vi "drive-auto.vi"() -> ()   [LabVIEW 2018]
doc: "This VI is called for each TeleOp packet received from the DS where the robot is not disabled. It is often used to read from the joysticks and update I/O or to update setpoints for timed control loops. It should complete and return within 20 milliseconds or it may miss DS packets."
uses:
  <vilib>/Rock Robotics/WPI/Solenoid/WPI_SolenoidValue.ctl
  <vilib>/Rock Robotics/WPI/ThirdParty/Phoenix-LabVIEW/Motor Controller/Controls/CTRE_Phoenix_MotorControl_ControlMode.ctl
  2e9e096c-a0d6-4374-a758-daa4b7bc34b9.vi
  069bde93-6a50-4702-a448-63a100da85ba.vi
  93fe4f39-d887-44e8-b42b-40b0db67de57.vi
  <vilib>/Rock Robotics/WPI/Utilities/WPI_GetSetVariantRefNum.vi
  <vilib>/Rock Robotics/Network Tables/NT Write Boolean Array.vi
  <vilib>/Rock Robotics/Network Tables/NT Write Numeric Array.vi
  Robot Global Data.vi
  <vilib>/Rock Robotics/WPI/Solenoid/WPI_SolenoidSetEnum.vi
  <vilib>/Rock Robotics/WPI/ThirdParty/Phoenix-LabVIEW/Motor Controller/Get/CTRE_Phoenix_MotorController_GetSelectedSensorData.vi
  <vilib>/Rock Robotics/WPI/ThirdParty/Phoenix-LabVIEW/Motor Controller/Get/CTRE_Phoenix_MotorController_GetOutputCurrent_Enhanced.vi
panel:
  out "Level":string="Low"
  out "GamePiece":string="Hatch"
  out "Output Voltage 4":dbl
  out "Output Voltage 3":dbl
  out "Output Voltage 2":dbl
  out "Output Voltage":dbl
  out "wrist sensor":i32
  out "Arm sensor":i32
  out "x output 2":dbl
  out "y output 2":dbl
  # "left"
  # "RIGHT"
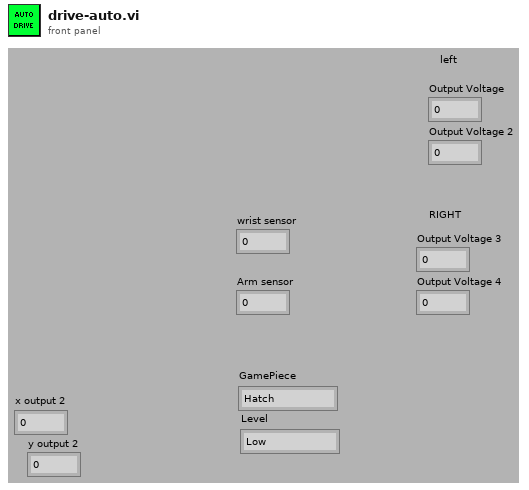
[diagram p1: front panel]
types:
  T1 = typedef "WPI_SolenoidValue.ctl" = enum16{"Off", "On", "Forward", "Reverse"}
  T2 = typedef "WPI_JoystickDevRef.ctl" = cluster{"Device":T3}
  T3 = typedef "WPI_JoystickDeviceEnum.ctl" = enum16{"USB 0", "USB 1", "USB 2", "USB 3", "USB 4", "USB 5"}
  T4 = typedef "WPI_RobotDriveDevRef.ctl" = cluster{"DevStatus":errorcluster, "Motors[]":T5[], "Square Inputs":bool, "Max Output":dbl}
  T5 = typedef "WPI_MotorControlDeviceRef.ctl" = cluster{"DeviceStatus":errorcluster, "Type":T6, "PWM":cluster{"PWM Channel":T7, "DeadBand":T8}, "CAN":cluster{"Device Number":u8, "SetOutput VI Ref":variant, "GetOutput VI Ref":variant, "Enable VI Ref":variant, "Disable VI Ref":variant, "Data":variant}, "Invert":bool, "DIO PWM":cluster{"PWM \"Enable\" Channel":T7, "DIOChannel":T9, "PWM Rate":dbl}}
  T6 = typedef "WPI_MotorControlType.ctl" = enum16{"PWM", "CAN", "DIO PWM"}
  T7 = typedef "FPGA_DIOPWMChannel.ctl" = enum8{"PWM 0", "PWM 1", "PWM 2", "PWM 3", "PWM 4", "PWM 5", "PWM 6", "PWM 7", "PWM 8", "PWM 9", "PWM MXP 0", "PWM MXP 1", "PWM MXP 2", "PWM MXP 3", "PWM MXP 4", "PWM MXP 5", "PWM MXP 6", "PWM MXP 7", "PWM MXP 8", "PWM MXP 9", "Invalid"}
  T8 = typedef "WPI_PWMDeadband.ctl" = cluster{"Name":string, "maxPositivePwm":i32, "minPositivePwm":i32, "centerPwm":i32, "maxNegativePwm":i32, "minNegativePwm":i32, "angularRange":u16}
  T9 = typedef "FPGA_DIOChannel.ctl" = enum8{"DIO 0", "DIO 1", "DIO 2", "DIO 3", "DIO 4", "DIO 5", "DIO 6", "DIO 7", "DIO 8", "DIO 9", "DIO MXP 0", "DIO MXP 1", "DIO MXP 2", "DIO MXP 3", "DIO MXP 4", "DIO MXP 5", "DIO MXP 6", "DIO MXP 7", "DIO MXP 8", "DIO MXP 9", "DIO MXP 10", "DIO MXP 11", "DIO MXP 12", "DIO MXP 13", "DIO MXP 14", "DIO MXP 15", "SPI Port CS1", "SPI Port CS2", "SPI Port CS3", "SPI Port MISO", "SPI Port MOSI", "Invalid"}
  T10 = typedef "WPI_SolenoidDevRef.ctl" = cluster{"DevStatus":errorcluster, "Pneumatics Control Module":u8, "Forward Solenoid Channel":T11, "Reverse Solenoid Channel":T11}
  T11 = typedef "WPI_SolenoidChannel.ctl" = enum8{"Solenoid 0", "Solenoid 1", "Solenoid 2", "Solenoid 3", "Solenoid 4", "Solenoid 5", "Solenoid 6", "Solenoid 7", "Invalid"}
  T12 = typedef "CTRE_Phoenix_MotorControl_ControlMode.ctl" = u16
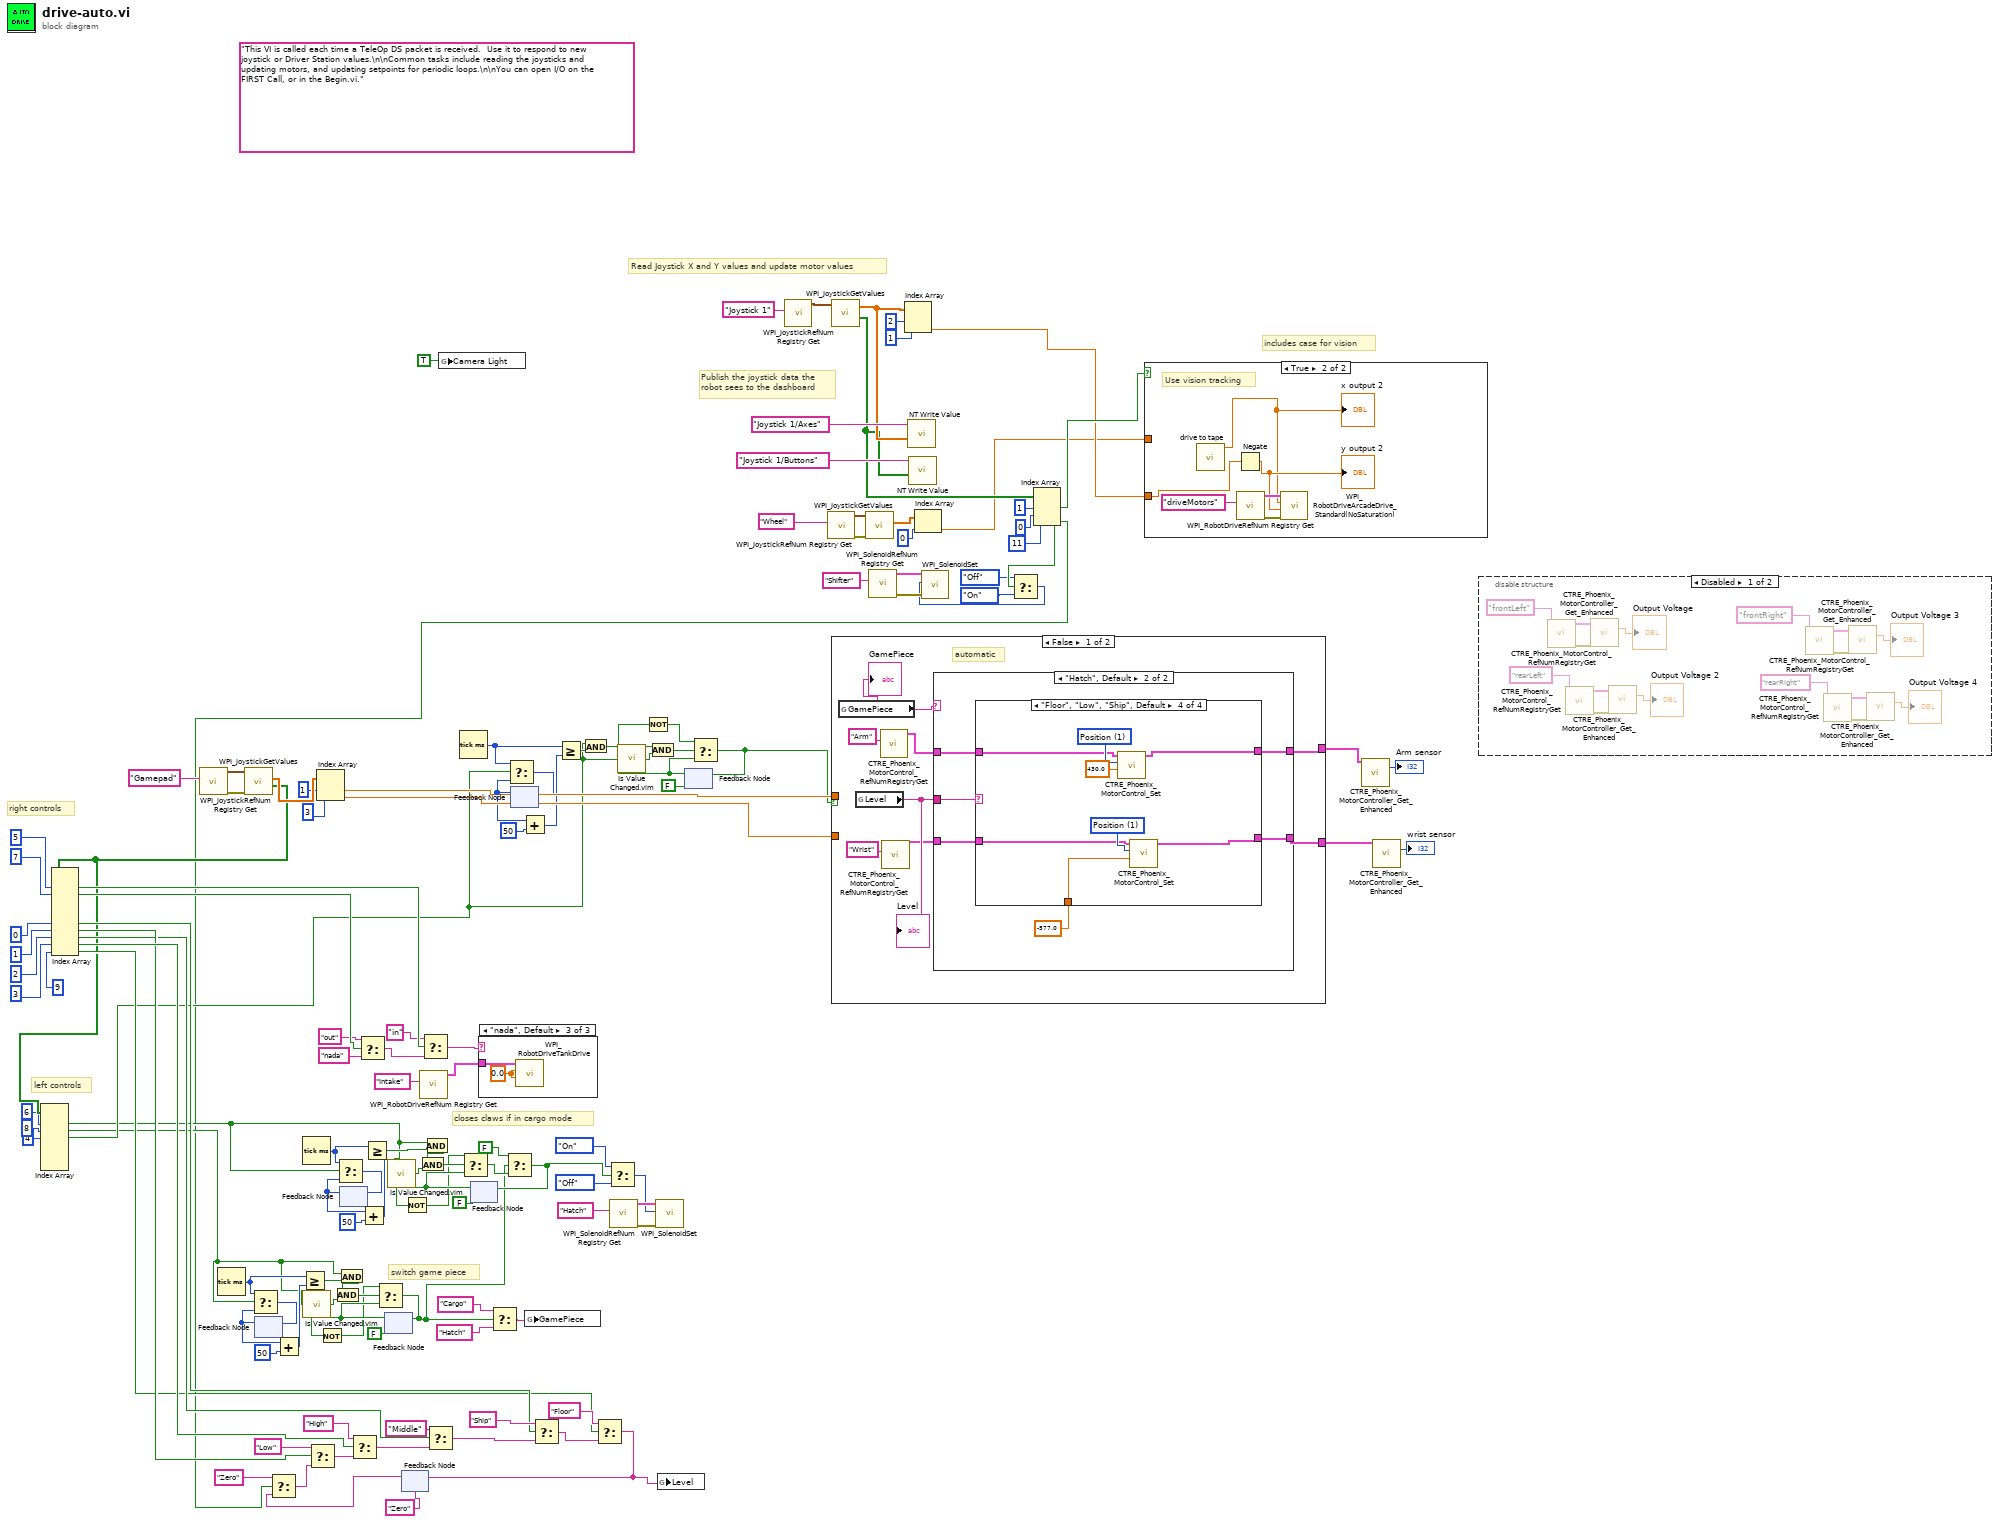
[diagram p0: block diagram]
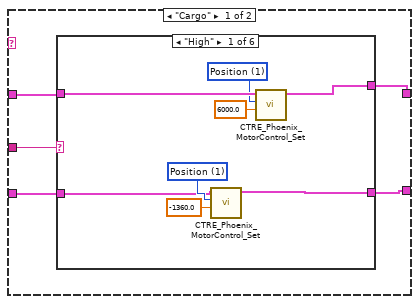
[diagram p3: hidden frame]
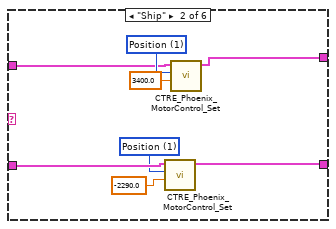
[diagram p4: hidden frame]
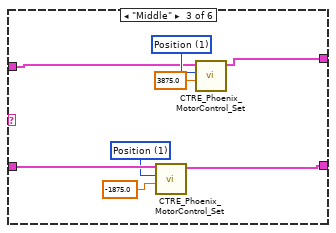
[diagram p5: hidden frame]
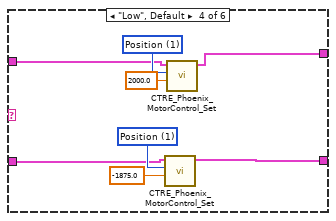
[diagram p6: hidden frame]
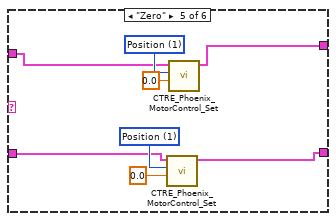
[diagram p7: hidden frame]
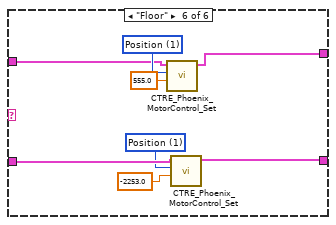
[diagram p8: hidden frame]
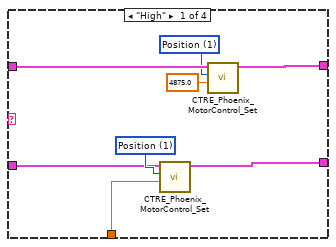
[diagram p9: hidden frame]
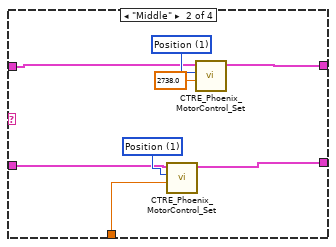
[diagram p10: hidden frame]
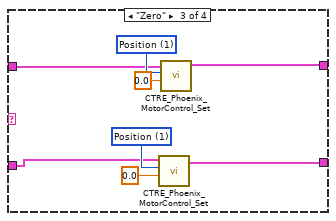
[diagram p11: hidden frame]
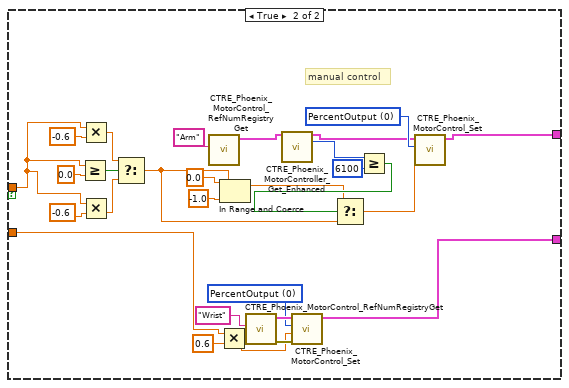
[diagram p12: hidden frame]
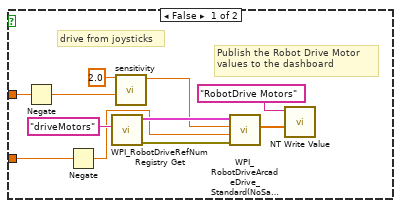
[diagram p13: hidden frame]
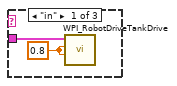
[diagram p14: hidden frame]
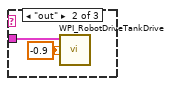
[diagram p15: hidden frame]
diagram:
  (unwired) "This VI is called each time a TeleOp DS packet is received.  Use it to respond to new joystick or Driver Station values.\n\nCommon tasks include reading the joysticks and updating motors, and updating setpoints for periodic loops.\n\nYou can open I/O on the FIRST Call, or in the Begin.vi."
  # "closes claws if in cargo mode"
  # "switch game piece"
  # "left controls"
  # "right controls"
  # "includes case for vision"
  # "Publish the joystick data the\nrobot sees to the dashboard"
  # "Read Joystick X and Y values and update motor values"
  n1 = call <vilib>:"WPI_JoystickRefNum Registry Get.vi"("refnum name"="Gamepad") -> ("error out"=w114:errorcluster, "JoystickDevRef"=w117:T2)  [unwired: 1 in, 8 out]
  n2 = Tick Count (ms)() -> (millisecond timer value=w49:u32)
  n3 = call <vilib>:"WPI_JoystickGetValues.vi"("error in (no error)"=w114, "JoystickDevRef"=w117) -> ("Buttons"=w18:bool[], "Axes"=w116:dbl[])  [unwired: 5 in, 3 out]
  n4 = Index Array(array=w18, index #1=6 ("index"), index #2=8 ("index"), index #3=4 ("index")) -> (element #1=w12:bool, element #2=w13:bool, element #3=w14:bool)  [unwired: 4 in, 4 out]
  n5 = Index Array(array=w18, index #1=5 ("index"), index #2=7 ("index"), index #6=0 ("index"), index #7=1 ("index"), index #8=2 ("index"), index #9=3 ("index"), index #10=9 ("index")) -> (element #1=w111:bool, element #2=w106:bool, element #6=w25:bool, element #7=w24:bool, element #8=w23:bool, element #9=w26:bool, element #10=w19:bool)  [unwired: 3 in, 3 out]
  n6 = feedback #1() -> (w40:u32)  [unwired: 1 in]
  n7 = Select(t=w49, s=w13, f=w40) -> (s? t:f=w47:u32)
  n8 = feedback-in #1(w47) -> ()
  n9 = Add(x=w40, y=u32 50) -> (x+y=w48:u32)
  n10 = Greater Or Equal?(x=w49, y=w48) -> (x >= y?=w50:bool)
  n11 = Tick Count (ms)() -> (millisecond timer value=w81:u32)
  n12 = call "Is Value Changed.vim"("value"=w13) -> ("changed or first call?"=w45:bool)
  n13 = Index Array(array=w116, index #1=1 ("index"), index #2=3 ("index")) -> (element #1=w70:dbl, element #2=w71:dbl)
  n14 = And(x=w13, y=w50) -> (x .and. y?=w51:bool)
  n15 = And(x=w51, y=w45) -> (x .and. y?=w44:bool)
  n16 = feedback #2() -> (w72:u32)  [unwired: 1 in]
  n17 = Select(t=w81, s=w12, f=w72) -> (s? t:f=w79:u32)
  n18 = feedback-in #2(w79) -> ()
  n19 = Select(t="out", s=w106, f="nada") -> (s? t:f=w107:string)
  n20 = Add(x=w72, y=u32 50) -> (x+y=w80:u32)
  n21 = Greater Or Equal?(x=w81, y=w80) -> (x >= y?=w82:bool)
  n22 = feedback #3(FALSE) -> (w43:bool)
  n23 = Not(x=w43) -> (.not. x?=w41:bool)
  n24 = Select(t=w41, s=w44, f=w43) -> (s? t:f=w2:bool)
  n25 = feedback-in #3(w2) -> ()
  n26 = call "Is Value Changed.vim"("value"=w12) -> ("changed or first call?"=w77:bool)
  n27 = feedback #4("Zero") -> (w9:string)
  n28 = call <vilib>:"WPI_RobotDriveRefNum Registry Get.vi"("refnum name"="Intake") -> ("RobotDriveDevRef"=w102:T4)  [unwired: 9 in, 1 out]
  n29 = Select(t="in", s=w111, f=w107) -> (s? t:f=w110:string)
  n30 = And(x=w12, y=w82) -> (x .and. y?=w83:bool)
  n31 = And(x=w83, y=w77) -> (x .and. y?=w76:bool)
  n32 = global write "Robot Global Data.vi" "Camera Light"(TRUE ("Camera Light")) -> ()
  n33 = Tick Count (ms)() -> (millisecond timer value=w67:u32)
  n34 = feedback #5(FALSE) -> (w75:bool)
  n35 = Not(x=w75) -> (.not. x?=w73:bool)
  n36 = Select(t=w73, s=w76, f=w75) -> (s? t:f=w3:bool)
  n37 = case shown="\"nada\", Default" w110 {
    tunnel: w102 -> [w133 w135 w137]
    frame "in" {
      w134 = 0.8
      n38 = call <vilib>:"WPI_RobotDriveTankDrive.vi"("Right axis value"=w134, "Left axis value"=w134, "RobotDriveDevRef"=w133) -> ()  [unwired: 6 in, 3 out]
    }
    frame "out" {
      w136 = -0.9
      n39 = call <vilib>:"WPI_RobotDriveTankDrive.vi"("Right axis value"=w136, "Left axis value"=w136, "RobotDriveDevRef"=w135) -> ()  [unwired: 6 in, 3 out]
    }
    frame "nada", Default {
      w138 = 0.0
      n40 = call <vilib>:"WPI_RobotDriveTankDrive.vi"("Right axis value"=w138, "Left axis value"=w138, "RobotDriveDevRef"=w137) -> ()  [unwired: 6 in, 3 out]
    }
  }
  n41 = Select(t="Cargo", s=w2, f="Hatch") -> (s? t:f=w53:string)
  n42 = Select(t=FALSE, s=w2, f=w3) -> (s? t:f=w4:bool)
  n43 = feedback-in #5(w4) -> ()
  n44 = feedback #6() -> (w58:u32)  [unwired: 1 in]
  n45 = Select(t=w67, s=w14, f=w58) -> (s? t:f=w65:u32)
  n46 = feedback-in #6(w65) -> ()
  n47 = Add(x=w58, y=u32 50) -> (x+y=w66:u32)
  n48 = global write "Robot Global Data.vi" "GamePiece"(w53) -> ()
  n49 = Greater Or Equal?(x=w67, y=w66) -> (x >= y?=w68:bool)
  n50 = And(x=w14, y=w68) -> (x .and. y?=w69:bool)
  n51 = Select(t=WPI_SolenoidValue."On" ("Value"), s=w4, f=WPI_SolenoidValue."Off") -> (s? t:f=w98:T1)
  n52 = call <vilib>:"WPI_SolenoidRefNum Registry Get.vi"("refnum name"="Hatch") -> ("error out"=w101:errorcluster, "SolenoidDevRef"=w100:T10)  [unwired: 9 in]
  n53 = call "Is Value Changed.vim"("value"=w14) -> ("changed or first call?"=w63:bool)
  n54 = And(x=w69, y=w63) -> (x .and. y?=w62:bool)
  n55 = call-poly <vilib>:"WPI_SolenoidSet.vi"("error in (no error)"=w101, "Value"=w98, "SolenoidDevRef"=w100) -> ()  [unwired: 7 in, 2 out]
  n56 = feedback #7(FALSE) -> (w61:bool)
  n57 = Not(x=w61) -> (.not. x?=w59:bool)
  n58 = Select(t=w59, s=w62, f=w61) -> (s? t:f=w57:bool)
  n59 = feedback-in #7(w57) -> ()
  n60 = call <vilib>:"WPI_JoystickRefNum Registry Get.vi"("refnum name"="Joystick 1") -> ("JoystickDevRef"=w131:T2)  [unwired: 1 in, 9 out]
  n61 = call <vilib>:"WPI_JoystickRefNum Registry Get.vi"("refnum name"="Wheel") -> ("error out"=w125:errorcluster, "JoystickDevRef"=w124:T2)  [unwired: 9 in]
  n62 = call <vilib>:"WPI_JoystickGetValues.vi"("JoystickDevRef"=w131) -> ("Buttons"=w120:bool[], "Axes"=w128:dbl[])  [unwired: 6 in, 3 out]
  n63 = case shown="False" w57 {
    tunnel: w71 -> [_ w258]
    tunnel: w70 -> [_ w250]
    tunnel: [w139 w249] -> w55
    tunnel: [w143 w248] -> w54
    frame False {
      # "automatic"
      n64 = global read "Robot Global Data.vi" "GamePiece"() -> (w142:string)
      "GamePiece" <- w142
      n65 = global read "Robot Global Data.vi" "Level"() -> (w141:string)
      "Level" <- w141
      n66 = call <vilib>:"CTRE_Phoenix_MotorControl_RefNumRegistryGet.vi"("refnum name"="Arm") -> ("PhoenixMotorControlDevRef"=w146:T5)  [unwired: 9 in, 1 out]
      n67 = call <vilib>:"CTRE_Phoenix_MotorControl_RefNumRegistryGet.vi"("refnum name"="Wrist") -> ("PhoenixMotorControlDevRef"=w140:T5)  [unwired: 9 in, 1 out]
      n68 = case shown="\"Hatch\", Default" w142 {
        tunnel: w146 -> [w150 w205]
        tunnel: [w151 w204] -> w143
        tunnel: [w149 w203] -> w139
        tunnel: w141 -> [w148 w202]
        tunnel: w140 -> [w147 w201]
        frame "Cargo" {
          n69 = case shown="\"High\"" w148 {
            tunnel: w150 -> [w159 w166 w174 w182 w187 w198]
            tunnel: [w157 w165 w173 w181 w186 w197] -> w151
            tunnel: [w155 w163 w171 w179 w185 w195] -> w149
            tunnel: w147 -> [w152 w162 w170 w176 w184 w194]
            frame "High" {
              w153 = T12 1 items=["PercentOutput"=0, "Position"=1, "Velocity"=2, "Current"=3, "Follower"=5, "MotionProfile"=6, "MotionMagic"=7, "MotionProfileArc"=10, "Disabled"=15] ("Control Mode")
              w158 = T12 1 items=["PercentOutput"=0, "Position"=1, "Velocity"=2, "Current"=3, "Follower"=5, "MotionProfile"=6, "MotionMagic"=7, "MotionProfileArc"=10, "Disabled"=15] ("Control Mode")
              n70 = call <vilib>:"CTRE_Phoenix_MotorControl_Set.vi"("Output"=-1360.0, "Control Mode"=w153, "PhoenixMotorControlDevRef"=w152) -> ("PhoenixMotorControlDevRef"=w155:T5)  [unwired: 7 in, 1 out]
              n71 = call <vilib>:"CTRE_Phoenix_MotorControl_Set.vi"("Output"=6000.0, "Control Mode"=w158, "PhoenixMotorControlDevRef"=w159) -> ("PhoenixMotorControlDevRef"=w157:T5)  [unwired: 7 in, 1 out]
            }
            frame "Ship" {
              w160 = T12 1 items=["PercentOutput"=0, "Position"=1, "Velocity"=2, "Current"=3, "Follower"=5, "MotionProfile"=6, "MotionMagic"=7, "MotionProfileArc"=10, "Disabled"=15] ("Control Mode")
              w167 = T12 1 items=["PercentOutput"=0, "Position"=1, "Velocity"=2, "Current"=3, "Follower"=5, "MotionProfile"=6, "MotionMagic"=7, "MotionProfileArc"=10, "Disabled"=15] ("Control Mode")
              n72 = call <vilib>:"CTRE_Phoenix_MotorControl_Set.vi"("Output"=-2290.0, "Control Mode"=w160, "PhoenixMotorControlDevRef"=w162) -> ("PhoenixMotorControlDevRef"=w163:T5)  [unwired: 7 in, 1 out]
              n73 = call <vilib>:"CTRE_Phoenix_MotorControl_Set.vi"("Output"=3400.0, "Control Mode"=w167, "PhoenixMotorControlDevRef"=w166) -> ("PhoenixMotorControlDevRef"=w165:T5)  [unwired: 7 in, 1 out]
            }
            frame "Middle" {
              w168 = T12 1 items=["PercentOutput"=0, "Position"=1, "Velocity"=2, "Current"=3, "Follower"=5, "MotionProfile"=6, "MotionMagic"=7, "MotionProfileArc"=10, "Disabled"=15] ("Control Mode")
              w175 = T12 1 items=["PercentOutput"=0, "Position"=1, "Velocity"=2, "Current"=3, "Follower"=5, "MotionProfile"=6, "MotionMagic"=7, "MotionProfileArc"=10, "Disabled"=15] ("Control Mode")
              n74 = call <vilib>:"CTRE_Phoenix_MotorControl_Set.vi"("Output"=-1875.0, "Control Mode"=w168, "PhoenixMotorControlDevRef"=w170) -> ("PhoenixMotorControlDevRef"=w171:T5)  [unwired: 7 in, 1 out]
              n75 = call <vilib>:"CTRE_Phoenix_MotorControl_Set.vi"("Output"=3875.0, "Control Mode"=w175, "PhoenixMotorControlDevRef"=w174) -> ("PhoenixMotorControlDevRef"=w173:T5)  [unwired: 7 in, 1 out]
            }
            frame "Low", Default {
              w177 = T12 1 items=["PercentOutput"=0, "Position"=1, "Velocity"=2, "Current"=3, "Follower"=5, "MotionProfile"=6, "MotionMagic"=7, "MotionProfileArc"=10, "Disabled"=15] ("Control Mode")
              w183 = T12 1 items=["PercentOutput"=0, "Position"=1, "Velocity"=2, "Current"=3, "Follower"=5, "MotionProfile"=6, "MotionMagic"=7, "MotionProfileArc"=10, "Disabled"=15] ("Control Mode")
              n76 = call <vilib>:"CTRE_Phoenix_MotorControl_Set.vi"("Output"=-1875.0, "Control Mode"=w177, "PhoenixMotorControlDevRef"=w176) -> ("PhoenixMotorControlDevRef"=w179:T5)  [unwired: 7 in, 1 out]
              n77 = call <vilib>:"CTRE_Phoenix_MotorControl_Set.vi"("Output"=2000.0, "Control Mode"=w183, "PhoenixMotorControlDevRef"=w182) -> ("PhoenixMotorControlDevRef"=w181:T5)  [unwired: 7 in, 1 out]
            }
            frame "Zero" {
              w188 = T12 1 items=["PercentOutput"=0, "Position"=1, "Velocity"=2, "Current"=3, "Follower"=5, "MotionProfile"=6, "MotionMagic"=7, "MotionProfileArc"=10, "Disabled"=15] ("Control Mode")
              w191 = T12 1 items=["PercentOutput"=0, "Position"=1, "Velocity"=2, "Current"=3, "Follower"=5, "MotionProfile"=6, "MotionMagic"=7, "MotionProfileArc"=10, "Disabled"=15] ("Control Mode")
              n78 = call <vilib>:"CTRE_Phoenix_MotorControl_Set.vi"("Output"=0.0, "Control Mode"=w188, "PhoenixMotorControlDevRef"=w184) -> ("PhoenixMotorControlDevRef"=w185:T5)  [unwired: 7 in, 1 out]
              n79 = call <vilib>:"CTRE_Phoenix_MotorControl_Set.vi"("Output"=0.0, "Control Mode"=w191, "PhoenixMotorControlDevRef"=w187) -> ("PhoenixMotorControlDevRef"=w186:T5)  [unwired: 7 in, 1 out]
            }
            frame "Floor" {
              w192 = T12 1 items=["PercentOutput"=0, "Position"=1, "Velocity"=2, "Current"=3, "Follower"=5, "MotionProfile"=6, "MotionMagic"=7, "MotionProfileArc"=10, "Disabled"=15] ("Control Mode")
              w199 = T12 1 items=["PercentOutput"=0, "Position"=1, "Velocity"=2, "Current"=3, "Follower"=5, "MotionProfile"=6, "MotionMagic"=7, "MotionProfileArc"=10, "Disabled"=15] ("Control Mode")
              n80 = call <vilib>:"CTRE_Phoenix_MotorControl_Set.vi"("Output"=555.0, "Control Mode"=w199, "PhoenixMotorControlDevRef"=w198) -> ("PhoenixMotorControlDevRef"=w197:T5)  [unwired: 7 in, 1 out]
              n81 = call <vilib>:"CTRE_Phoenix_MotorControl_Set.vi"("Output"=-2253.0, "Control Mode"=w192, "PhoenixMotorControlDevRef"=w194) -> ("PhoenixMotorControlDevRef"=w195:T5)  [unwired: 7 in, 1 out]
            }
          }
        }
        frame "Hatch", Default {
          n82 = case shown="\"Floor\", \"Low\", \"Ship\", Default" w202 {
            tunnel: w205 -> [w213 w220 w225 w236]
            tunnel: [w211 w219 w224 w235] -> w204
            tunnel: [w209 w217 w223 w233] -> w203
            tunnel: w201 -> [w207 w215 w222 w231]
            tunnel: -577.0 ("Output") -> [w206 w214 _ w230]
            frame "High" {
              w208 = T12 1 items=["PercentOutput"=0, "Position"=1, "Velocity"=2, "Current"=3, "Follower"=5, "MotionProfile"=6, "MotionMagic"=7, "MotionProfileArc"=10, "Disabled"=15] ("Control Mode")
              w212 = T12 1 items=["PercentOutput"=0, "Position"=1, "Velocity"=2, "Current"=3, "Follower"=5, "MotionProfile"=6, "MotionMagic"=7, "MotionProfileArc"=10, "Disabled"=15] ("Control Mode")
              n83 = call <vilib>:"CTRE_Phoenix_MotorControl_Set.vi"("Output"=w206, "Control Mode"=w208, "PhoenixMotorControlDevRef"=w207) -> ("PhoenixMotorControlDevRef"=w209:T5)  [unwired: 7 in, 1 out]
              n84 = call <vilib>:"CTRE_Phoenix_MotorControl_Set.vi"("Output"=4875.0, "Control Mode"=w212, "PhoenixMotorControlDevRef"=w213) -> ("PhoenixMotorControlDevRef"=w211:T5)  [unwired: 7 in, 1 out]
            }
            frame "Middle" {
              w216 = T12 1 items=["PercentOutput"=0, "Position"=1, "Velocity"=2, "Current"=3, "Follower"=5, "MotionProfile"=6, "MotionMagic"=7, "MotionProfileArc"=10, "Disabled"=15] ("Control Mode")
              w221 = T12 1 items=["PercentOutput"=0, "Position"=1, "Velocity"=2, "Current"=3, "Follower"=5, "MotionProfile"=6, "MotionMagic"=7, "MotionProfileArc"=10, "Disabled"=15] ("Control Mode")
              n85 = call <vilib>:"CTRE_Phoenix_MotorControl_Set.vi"("Output"=w214, "Control Mode"=w216, "PhoenixMotorControlDevRef"=w215) -> ("PhoenixMotorControlDevRef"=w217:T5)  [unwired: 7 in, 1 out]
              n86 = call <vilib>:"CTRE_Phoenix_MotorControl_Set.vi"("Output"=2738.0, "Control Mode"=w221, "PhoenixMotorControlDevRef"=w220) -> ("PhoenixMotorControlDevRef"=w219:T5)  [unwired: 7 in, 1 out]
            }
            frame "Zero" {
              w226 = T12 1 items=["PercentOutput"=0, "Position"=1, "Velocity"=2, "Current"=3, "Follower"=5, "MotionProfile"=6, "MotionMagic"=7, "MotionProfileArc"=10, "Disabled"=15] ("Control Mode")
              w229 = T12 1 items=["PercentOutput"=0, "Position"=1, "Velocity"=2, "Current"=3, "Follower"=5, "MotionProfile"=6, "MotionMagic"=7, "MotionProfileArc"=10, "Disabled"=15] ("Control Mode")
              n87 = call <vilib>:"CTRE_Phoenix_MotorControl_Set.vi"("Output"=0.0, "Control Mode"=w226, "PhoenixMotorControlDevRef"=w222) -> ("PhoenixMotorControlDevRef"=w223:T5)  [unwired: 7 in, 1 out]
              n88 = call <vilib>:"CTRE_Phoenix_MotorControl_Set.vi"("Output"=0.0, "Control Mode"=w229, "PhoenixMotorControlDevRef"=w225) -> ("PhoenixMotorControlDevRef"=w224:T5)  [unwired: 7 in, 1 out]
            }
            frame "Floor", "Low", "Ship", Default {
              w232 = T12 1 items=["PercentOutput"=0, "Position"=1, "Velocity"=2, "Current"=3, "Follower"=5, "MotionProfile"=6, "MotionMagic"=7, "MotionProfileArc"=10, "Disabled"=15] ("Control Mode")
              w237 = T12 1 items=["PercentOutput"=0, "Position"=1, "Velocity"=2, "Current"=3, "Follower"=5, "MotionProfile"=6, "MotionMagic"=7, "MotionProfileArc"=10, "Disabled"=15] ("Control Mode")
              n89 = call <vilib>:"CTRE_Phoenix_MotorControl_Set.vi"("Output"=430.0, "Control Mode"=w237, "PhoenixMotorControlDevRef"=w236) -> ("PhoenixMotorControlDevRef"=w235:T5)  [unwired: 7 in, 1 out]
              n90 = call <vilib>:"CTRE_Phoenix_MotorControl_Set.vi"("Output"=w230, "Control Mode"=w232, "PhoenixMotorControlDevRef"=w231) -> ("PhoenixMotorControlDevRef"=w233:T5)  [unwired: 7 in, 1 out]
            }
          }
        }
      }
    }
    frame True {
      w261 = T12 0 items=["PercentOutput"=0, "Position"=1, "Velocity"=2, "Current"=3, "Follower"=5, "MotionProfile"=6, "MotionMagic"=7, "MotionProfileArc"=10, "Disabled"=15] ("Control Mode")
      w265 = T12 0 items=["PercentOutput"=0, "Position"=1, "Velocity"=2, "Current"=3, "Follower"=5, "MotionProfile"=6, "MotionMagic"=7, "MotionProfileArc"=10, "Disabled"=15] ("Control Mode")
      # "manual control"
      n91 = Greater Or Equal?(x=w250, y=0.0) -> (x >= y?=w256:bool)
      n92 = Multiply(x=w250, y=-0.6) -> (x*y=w251:dbl)
      n93 = Multiply(x=w250, y=-0.6) -> (x*y=w255:dbl)
      n94 = Select(t=w251, s=w256, f=w255) -> (s? t:f=w242:dbl)
      n95 = call <vilib>:"CTRE_Phoenix_MotorControl_RefNumRegistryGet.vi"("refnum name"="Arm") -> ("PhoenixMotorControlDevRef"=w246:T5)  [unwired: 9 in, 1 out]
      n96 = Multiply(x=w258, y=0.6) -> (x*y=w259:dbl)
      n97 = In Range and Coerce(upper limit=0.0, x=w242, lower limit=-1.0) -> (coerced(x)=w238:dbl)  [unwired: 1 out]
      n98 = call <vilib>:"CTRE_Phoenix_MotorControl_RefNumRegistryGet.vi"("refnum name"="Wrist") -> ("error out"=w263:errorcluster, "PhoenixMotorControlDevRef"=w262:T5)  [unwired: 9 in]
      n99 = call-poly <vilib>:"CTRE_Phoenix_MotorController_Get_Enhanced.vi"("PhoenixMotorControlDevRef"=w246) -> ("PhoenixMotorControlDevRef"=w247:T5, "Position (Raw Sensor Units)"=w245:i32)  [unwired: 11 in, 2 out]
      n100 = call <vilib>:"CTRE_Phoenix_MotorControl_Set.vi"("error in (no error)"=w263, "Output"=w259, "Control Mode"=w261, "PhoenixMotorControlDevRef"=w262) -> ("PhoenixMotorControlDevRef"=w249:T5)  [unwired: 6 in, 1 out]
      n101 = Greater Or Equal?(x=w245, y=6100) -> (x >= y?=w243:bool)
      n102 = Select(t=w238, s=w243, f=w242) -> (s? t:f=w239:dbl)
      n103 = call <vilib>:"CTRE_Phoenix_MotorControl_Set.vi"("Output"=w239, "Control Mode"=w265, "PhoenixMotorControlDevRef"=w247) -> ("PhoenixMotorControlDevRef"=w248:T5)  [unwired: 7 in, 1 out]
    }
  }
  n104 = call <vilib>:"WPI_JoystickGetValues.vi"("error in (no error)"=w125, "JoystickDevRef"=w124) -> ("Axes"=w123:dbl[])  [unwired: 5 in, 4 out]
  n105 = call <vilib>:"WPI_SolenoidRefNum Registry Get.vi"("refnum name"="Shifter") -> ("error out"=w94:errorcluster, "SolenoidDevRef"=w93:T10)  [unwired: 9 in]
  n106 = Index Array(array=w128, index #1=2 ("index"), index #2=1 ("index")) -> (element #2=w85:dbl)  [unwired: 1 out]
  n107 = call-poly <vilib>:"NT Write Value.vi"("Numeric Array"=w128, "Name"="Joystick 1/Axes") -> ()  [unwired: 9 in, 1 out]
  n108 = call-poly <vilib>:"NT Write Value.vi"("Boolean Array"=w120, "Name"="Joystick 1/Buttons") -> ()  [unwired: 9 in, 1 out]
  n109 = Index Array(array=w123, index=0) -> (element=w84:dbl)
  n110 = Index Array(array=w120, index #1=1 ("index"), index #2=0 ("index"), index #3=11 ("index")) -> (element #1=w86:bool, element #2=w91:bool, element #3=w6:bool)
  n111 = Select(t="Zero", s=w6, f=w9) -> (s? t:f=w5:string)
  n112 = Select(t="Low", s=w24, f=w5) -> (s? t:f=w31:string)
  n113 = Select(t="High", s=w26, f=w31) -> (s? t:f=w30:string)
  n114 = Select(t="Middle", s=w23, f=w30) -> (s? t:f=w28:string)
  n115 = Select(t="Ship", s=w25, f=w28) -> (s? t:f=w20:string)
  n116 = Select(t="Floor", s=w19, f=w20) -> (s? t:f=w22:string)
  n117 = feedback-in #4(w22) -> ()
  n118 = global write "Robot Global Data.vi" "Level"(w22) -> ()
  n119 = Select(t=WPI_SolenoidValue."Off" ("Value"), s=w91, f=WPI_SolenoidValue."On" ("Value")) -> (s? t:f=w90:T1)
  n120 = call-poly <vilib>:"WPI_SolenoidSet.vi"("error in (no error)"=w94, "Value"=w90, "SolenoidDevRef"=w93) -> ()  [unwired: 7 in, 2 out]
  n121 = case shown="True" w86 {
    tunnel: w85 -> [w272 w277]
    tunnel: w84 -> [w271 _]
    frame False {
      # "drive from joysticks"
      # "Publish the Robot Drive Motor\nvalues to the dashboard"
      n122 = Negate(x=w271) -> (-x=w268:dbl)
      n123 = Negate(x=w272) -> (-x=w269:dbl)
      n124 = call <vilib>:"WPI_RobotDriveRefNum Registry Get.vi"("refnum name"="driveMotors") -> ("error out"=w270:errorcluster, "RobotDriveDevRef"=w275:T4)  [unwired: 1 in, 8 out]
      n125 = call "sensitivity.vi"("x"=w268, "sensitivity"=2.0) -> ("scaled value"=w267:dbl)  [unwired: 9 in]
      n126 = call <vilib>:"WPI_RobotDriveArcadeDrive_Standard(NoSaturation).vi"("error in (no error)"=w270, "Y axis value"=w269, "X axis value"=w267, "RobotDriveDevRef"=w275) -> ("Motor Values"=w276:dbl[])  [unwired: 7 out]
      n127 = call-poly <vilib>:"NT Write Value.vi"("Numeric Array"=w276, "Name"="RobotDrive Motors") -> ()  [unwired: 9 in, 1 out]
    }
    frame True {
      # "Use vision tracking"
      n128 = call "drive to tape.vi"() -> ("x output"=w278:dbl)  [unwired: 10 in, 1 out]
      "x output 2" <- w278
      n129 = Negate(x=w277) -> (-x=w279:dbl)
      "y output 2" <- w279
      n130 = call <vilib>:"WPI_RobotDriveRefNum Registry Get.vi"("refnum name"="driveMotors") -> ("error out"=w280:errorcluster, "RobotDriveDevRef"=w281:T4)  [unwired: 1 in, 8 out]
      n131 = call <vilib>:"WPI_RobotDriveArcadeDrive_Standard(NoSaturation).vi"("error in (no error)"=w280, "Y axis value"=w279, "X axis value"=w278, "RobotDriveDevRef"=w281) -> ()  [unwired: 8 out]
    }
  }
  n132 = call-poly <vilib>:"CTRE_Phoenix_MotorController_Get_Enhanced.vi"("PhoenixMotorControlDevRef"=w54) -> ("Position (Raw Sensor Units)"=→"Arm sensor":i32)  [unwired: 11 in, 3 out]
  n133 = call-poly <vilib>:"CTRE_Phoenix_MotorController_Get_Enhanced.vi"("PhoenixMotorControlDevRef"=w55) -> ("Position (Raw Sensor Units)"=→"wrist sensor":i32)  [unwired: 11 in, 3 out]
  n134 = disable-structure shown="Disabled" {
    frame Disabled {
      n135 = call <vilib>:"CTRE_Phoenix_MotorControl_RefNumRegistryGet.vi"("refnum name"="frontLeft") -> ("error out"=w297:errorcluster, "PhoenixMotorControlDevRef"=w298:T5)  [unwired: 9 in]
      n136 = call <vilib>:"CTRE_Phoenix_MotorControl_RefNumRegistryGet.vi"("refnum name"="rearLeft") -> ("error out"=w294:errorcluster, "PhoenixMotorControlDevRef"=w295:T5)  [unwired: 9 in]
      n137 = call-poly <vilib>:"CTRE_Phoenix_MotorController_Get_Enhanced.vi"("PhoenixMotorControlDevRef"=w298, "error in"=w297) -> ("Output Current"=→"Output Voltage":dbl)  [unwired: 11 in, 2 out]
      n138 = call-poly <vilib>:"CTRE_Phoenix_MotorController_Get_Enhanced.vi"("PhoenixMotorControlDevRef"=w295, "error in"=w294) -> ("Output Current"=→"Output Voltage 2":dbl)  [unwired: 11 in, 2 out]
      n139 = call <vilib>:"CTRE_Phoenix_MotorControl_RefNumRegistryGet.vi"("refnum name"="frontRight") -> ("error out"=w291:errorcluster, "PhoenixMotorControlDevRef"=w292:T5)  [unwired: 9 in]
      n140 = call <vilib>:"CTRE_Phoenix_MotorControl_RefNumRegistryGet.vi"("refnum name"="rearRight") -> ("error out"=w288:errorcluster, "PhoenixMotorControlDevRef"=w289:T5)  [unwired: 9 in]
      n141 = call-poly <vilib>:"CTRE_Phoenix_MotorController_Get_Enhanced.vi"("PhoenixMotorControlDevRef"=w292, "error in"=w291) -> ("Output Current"=→"Output Voltage 3":dbl)  [unwired: 11 in, 2 out]
      n142 = call-poly <vilib>:"CTRE_Phoenix_MotorController_Get_Enhanced.vi"("PhoenixMotorControlDevRef"=w289, "error in"=w288) -> ("Output Current"=→"Output Voltage 4":dbl)  [unwired: 11 in, 2 out]
    }
    frame Enabled {
    }
  }
